vi "Real_float_to_double_word.vi"(4 "Real float":sgl=0.123456 min=0 format="%.6f") -> (0 "Seconda word":u16, 2 "Prima word":u16)   [LabVIEW 2022 SP3]
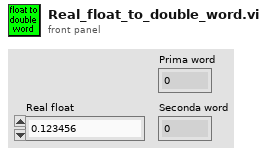
[diagram p1: front panel]
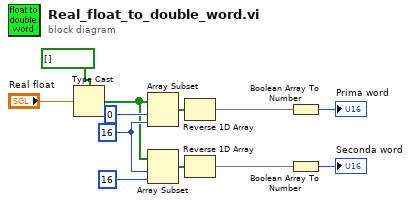
[diagram p0: block diagram]
diagram:
  w9 = 16 ("length")
  n1 = Type Cast(type=bool[] [], x="Real float") -> (*(type *) &x=w8:bool[])
  n2 = Array Subset(array=w8, index=0, length=w9) -> (w6:bool[])
  n3 = Array Subset(array=w8, index=w9, length=16) -> (w7:bool[])
  n4 = Reverse 1D Array(array=w6) -> (reversed array=w4:bool[])
  n5 = Reverse 1D Array(array=w7) -> (reversed array=w3:bool[])
  n6 = Boolean Array To Number(Boolean array=w4) -> (number=→"Prima word":u32)
  n7 = Boolean Array To Number(Boolean array=w3) -> (number=→"Seconda word":u32)
